vi "Internal_Point_Create_double.vi"(0 "Internal Map (variant)":variant, 5 "Tag Name":string, 11 "error in (no error)":errorcluster) -> (4 "Internal Map Out (variant)":variant, 6 "Tag Out":string, 10 "Point":T1, 14 "Datatype":T2=enum."double", 15 "error out":errorcluster)   [LabVIEW 2017, in "PointValueMap.lvlib"]
uses:
  <vilib>/addons/PointValueMap/PointValueMap.lvlib
  <vilib>/addons/PointValueMap/controls/DataTypes.ctl
  <vilib>/addons/PointValueMap/controls/Point.ctl
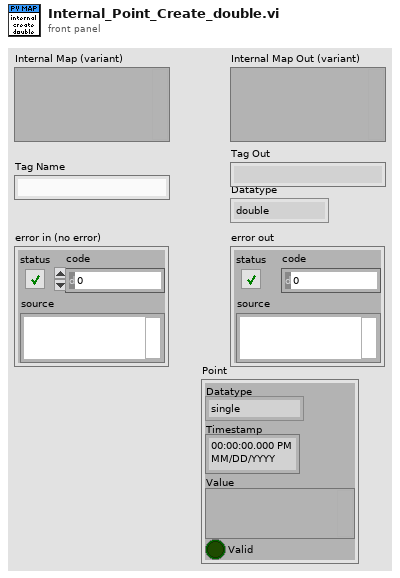
[diagram p1: front panel]
types:
  T1 = typedef "PointValueMap.lvlib/Point.ctl" = cluster{"Datatype":T2, "Timestamp":timestamp, "Value":variant, "Valid":bool}
  T2 = typedef "PointValueMap.lvlib/DataTypes.ctl" = enum16{"single", "double", "i32", "string", "variant"}
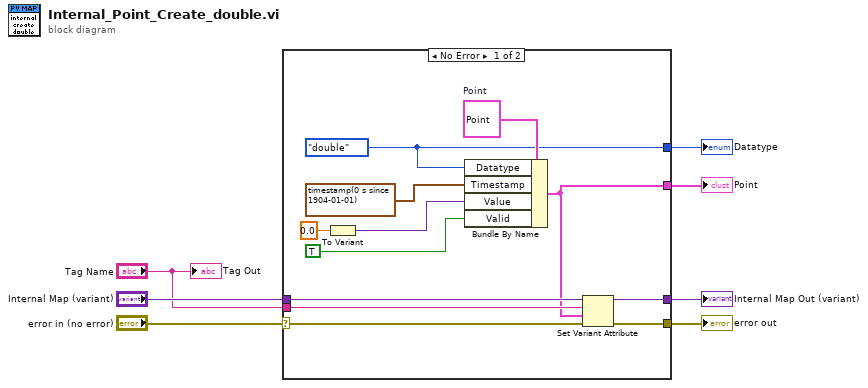
[diagram p0: block diagram]
diagram:
  n1 = case shown="No Error" "error in (no error)" {
    selector: "error in (no error)" -> [w13 w20]
    tunnel: "Internal Map (variant)" -> [w15 w21]
    tunnel: [w12 w20] -> w6
    tunnel: [w11 w21] -> w5
    tunnel: "Tag Name" -> [w14 _]
    tunnel: [w10 _] -> w2
    tunnel: [w9 _] -> w1
    frame No Error {
      w10 = DataTypes."double" ("Datatype")
      w19 = T1 {"Datatype"=enum."single", "Timestamp"=timestamp(0 s since 1904-01-01), "Value"=variant, "Valid"=FALSE}  # Point
      n2 = To Variant(anything=0.0) -> (Variant=w16:variant)
      n3 = Bundle By Name(cluster=w19, "Datatype"=w10, "Timestamp"=timestamp(0 s since 1904-01-01), "Value"=w16, "Valid"=TRUE) -> (w9:T1)
      n4 = Set Variant Attribute(Variant=w15, name=w14, value=w9, error in=w13) -> (Variant out=w11:variant, error out=w12:errorcluster)  [unwired: 1 out]
    }
    frame Error {
    }
  }
  "error out" <- w6
  "Internal Map Out (variant)" <- w5
  "Datatype" <- w2
  "Point" <- w1
  "Tag Out" <- "Tag Name"
